vi "Read value.vi"(8 "error in (no error)":errorcluster, 11 "UserDefinedWaveform in":refnum<class "UserDefinedWaveform.lvclass">) -> (0 "error out":errorcluster, 2 "value":string, 3 "UserDefinedWaveform out":refnum<class "UserDefinedWaveform.lvclass">)   [LabVIEW 2014, in "UserDefinedWaveform.lvclass"]
uses:
  UserDefinedWaveform.lvclass
  UserDefinedWaveform.lvclass/UserDefinedWaveform.ctl
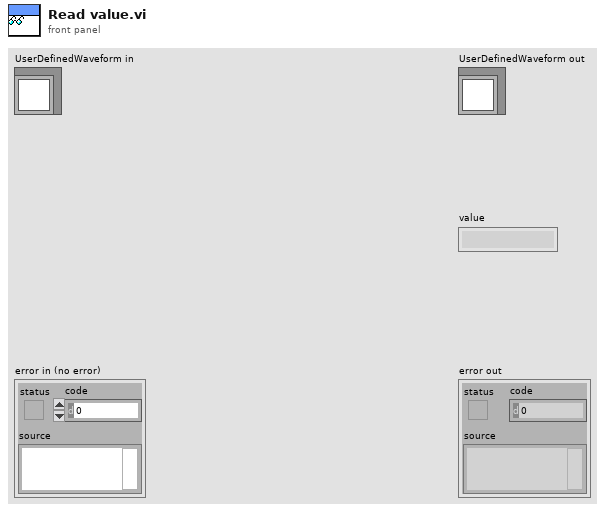
[diagram p1: front panel]
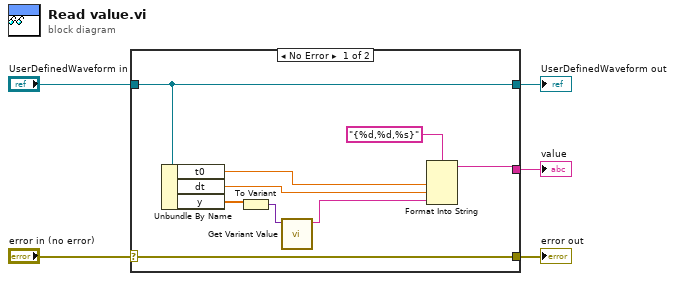
[diagram p0: block diagram]
diagram:
  n1 = case shown="No Error" "error in (no error)" {
    selector: "error in (no error)" -> [w14 w15]
    tunnel: [w14 w15] -> w4
    tunnel: [w13 w16] -> w2
    tunnel: "UserDefinedWaveform in" -> [w13 w16]
    tunnel: [w12 _] -> w1
    frame No Error {
      n2 = Unbundle By Name(w13) -> ("t0"=w11:dbl, "dt"=w10:dbl, "y"=w8:dbl[])
      n3 = To Variant(anything=w8) -> (Variant=w7:variant)
      n4 = call "Get Variant Value.vi"("Variant in"=w7) -> ("Variant value as string"=w6:string)  [unwired: 10 in]
      n5 = Format Into String(format string="{%d,%d,%s}", w11, w10, w6) -> (resulting string=w12:string)  [unwired: 2 in, 1 out]
    }
    frame Error {
    }
  }
  "error out" <- w4
  "UserDefinedWaveform out" <- w2
  "value" <- w1
